vi "connect.vi"(8 "error in (no error)":errorcluster, 10 "Database Path":path) -> (0 "error out":errorcluster, 3 "object out":refnum<class "SQLiteConnection.lvclass">)   [LabVIEW 2019, in "SQLiteConnection.lvclass"]
uses:
  SQLiteConnection.lvclass
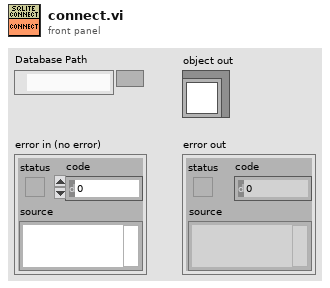
[diagram p1: front panel]
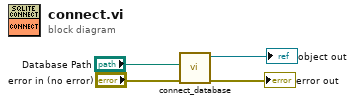
[diagram p0: block diagram]
diagram:
  n1 = call "connect_database.vi"("error in (no error)"="error in (no error)", "Database Path"="Database Path") -> ("error out"=→"error out":errorcluster, "object out"=→"object out":refnum<class "SQLiteConnection.lvclass">)  [unwired: 8 in]
